vi "Delete Empty Lines.vi"(1 "String":string) -> (0 "delimited string":string)   [LabVIEW 2019, in "Git.lvclass"]
uses:
  Git.lvclass
  <userlib>/_OpenG.lib/string/string.llb/Trim Whitespace (String)__ogtk.vi
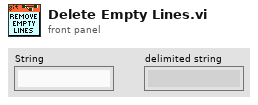
[diagram p1: front panel]
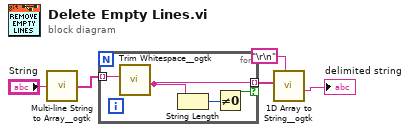
[diagram p0: block diagram]
diagram:
  n1 = call <userlib>:"Multi-line String to Array__ogtk.vi"("string"="String") -> ("lines"=w1:string[])
  n2 = for {
    tunnel: w1 -> [w9] mode=indexing
    tunnel: [w8] -> w2 mode=indexing if=w6
    n3 = call-poly <userlib>:"Trim Whitespace__ogtk.vi"("String in"=w9) -> ("String out"=w8:string)  [unwired: 6 in]
    n4 = String Length(string=w8) -> (length=w7:i32)
    n5 = Not Equal To 0?(x=w7) -> (x != 0?=w6:bool)
  }
  n6 = call <userlib>:"1D Array to String__ogtk.vi"("delimiter (Tab)"="\r\n", "Array of Strings"=w2) -> ("delimited string"=→"delimited string":string)  [unwired: 9 in]
